vi "WPI_RobotMotorDelayAndUpdateSafety.vi"(6 "Feed time (s)":dbl=0.05, 8 "error in (no error)":errorcluster, 10 "Delay (s)":dbl, 11 "MotorControlDevRef":T1={"DeviceStatus"={"status"=FALSE, "code"=0, "source"=""}, "Type"=enum."PWM", "PWM"={"Digital Module"=enum."Digital Module 1", "PWM Channel"=enum."Invalid", "DeadBand"={"Name"="", "maxPositivePwm"=0, "minPositivePwm"=0, "centerPwm"=0, "maxNegativePwm"=0, "minNegativePwm"=0, "angularRange"=0}}, "CAN"={"Device Number"=0, "Control Mode"=enum."Percent VBus", "Semaphore"=refnum, "Max Vout"=12.0}, "Invert"=FALSE, "TransformRef"=refnum, "InvTransformRef"=refnum}) -> (0 "error out":errorcluster, 3 "MotorControlDevRef 2":T1={"DeviceStatus"={"status"=FALSE, "code"=0, "source"=""}, "Type"=enum."PWM", "PWM"={"Digital Module"=enum."Digital Module 1", "PWM Channel"=enum."Invalid", "DeadBand"={"Name"="", "maxPositivePwm"=0, "minPositivePwm"=0, "centerPwm"=0, "maxNegativePwm"=0, "minNegativePwm"=0, "angularRange"=0}}, "CAN"={"Device Number"=0, "Control Mode"=enum."Percent VBus", "Semaphore"=refnum, "Max Vout"=12.0}, "Invert"=FALSE, "TransformRef"=refnum, "InvTransformRef"=refnum})   [LabVIEW 2012]
doc: "During autonomous, it is often useful to update motor speed, then delay before updating them again. This delay uses the refnum to easily sequence the operations, and it updates the safety mechanism so that the drive motors are not disabled.\n\nThis software is licensed. Open the labview\\readme\\WPI Robotics Library Open Source License.txt file for more information."
uses:
  <vilib>/Rock Robotics/WPI/MotorControl/WPI_MotorControlDeviceRef.ctl
  <vilib>/Rock Robotics/SystemInterfaces/Typedef/FPGA_TypedefDigitalModule.ctl
  <vilib>/Rock Robotics/SystemInterfaces/DIO/FPGA_DIOPWMChannel.ctl
  <vilib>/Rock Robotics/WPI/PWM/WPI_PWMDeadband.ctl
  <vilib>/Rock Robotics/WPI/CAN/Jaguar/SubVIs/WPI_CANJaguar_ControlMode.ctl
  <vilib>/Rock Robotics/WPI/PWM/WPI_PWMTransform_ConPane.ctl
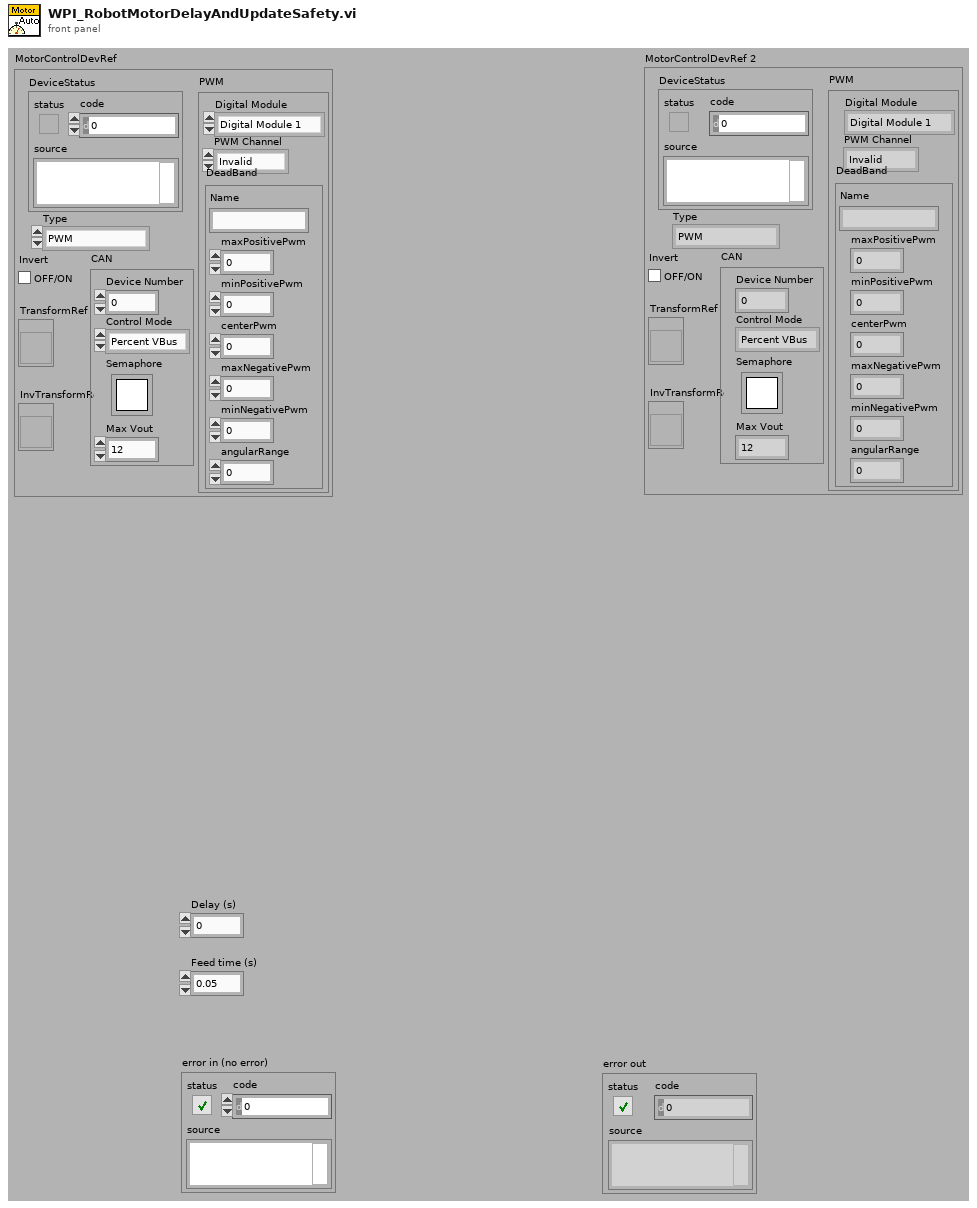
[diagram p1: front panel]
types:
  T1 = typedef "WPI_MotorControlDeviceRef.ctl" = cluster{"DeviceStatus":errorcluster, "Type":enum16{"PWM", "CAN"}, "PWM":cluster{"Digital Module":T2, "PWM Channel":T3, "DeadBand":T4}, "CAN":cluster{"Device Number":u8, "Control Mode":T5, "Semaphore":T6, "Max Vout":dbl}, "Invert":bool, "TransformRef":T7, "InvTransformRef":T7}
  T2 = typedef "FPGA_TypedefDigitalModule.ctl" = enum16{"Digital Module 1", "Digital Module 2"}
  T3 = typedef "FPGA_DIOPWMChannel.ctl" = enum8{"PWM 1", "PWM 2", "PWM 3", "PWM 4", "PWM 5", "PWM 6", "PWM 7", "PWM 8", "PWM 9", "PWM 10", "Invalid"}
  T4 = typedef "WPI_PWMDeadband.ctl" = cluster{"Name":string, "maxPositivePwm":i32, "minPositivePwm":i32, "centerPwm":i32, "maxNegativePwm":i32, "minNegativePwm":i32, "angularRange":u16}
  T5 = typedef "WPI_CANJaguar_ControlMode.ctl" = enum8{"Percent VBus", "Current", "Speed", "Position", "Voltage"}
  T6 = typedef "Semaphore RefNum" = refnum<k1>
  T7 = typedef "WPI_PWMTransform_ConPane.ctl" = refnum<vi>
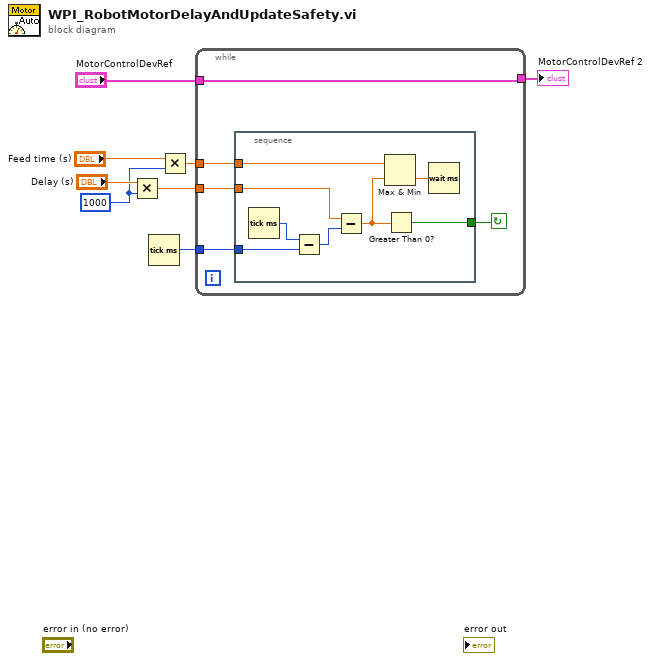
[diagram p0: block diagram]
diagram:
  w3 = 1000
  n1 = Multiply(x="Delay (s)", y=w3) -> (x*y=w6:dbl)
  n2 = Tick Count (ms)() -> (millisecond timer value=w8:u32)
  n3 = Multiply(x="Feed time (s)", y=w3) -> (x*y=w7:dbl)
  n4 = while {
    tunnel: w6 -> [w11]
    tunnel: [w9] -> w1
    tunnel: w7 -> [w12]
    tunnel: w8 -> [w13]
    tunnel: "MotorControlDevRef" -> [w9]
    stop <- w10 continue-if-true
    n5 = stacked-sequence {
      tunnel: w13 -> [w21]
      tunnel: w12 -> [w20]
      tunnel: w11 -> [w18]
      tunnel: [w14] -> w10
      frame #0 {
        n6 = Tick Count (ms)() -> (millisecond timer value=w16:u32)
        n7 = Subtract(x=w16, y=w21) -> (x-y=w17:u32)
        n8 = Subtract(x=w18, y=w17) -> (x-y=w15:dbl)
        n9 = Max & Min(x=w20, y=w15) -> (min(x,y)=w19:dbl)  [unwired: 1 out]
        n10 = Greater Than 0?(x=w15) -> (x > 0?=w14:bool)
        n11 = Wait (ms)(milliseconds to wait=w19) -> ()  [unwired: 1 out]
      }
    }
  }
  "MotorControlDevRef 2" <- w1
